vi "Notify Subscribers.vi"(8 "error in (no error)":errorcluster, 9 "Publish Time":timestamp, 10 "Topic Data":variant, 11 "Topic in":refnum<class "Topic.lvclass">) -> (0 "error out":errorcluster, 3 "Topic out":refnum<class "Topic.lvclass">)   [LabVIEW 2015, in "Mediator.lvlib" / "Topic.lvclass"]
doc: "<License>\nCopyright © 2017 Composed Systems, LLC | All rights reserved\nwww.composed.io\n\nAuthor: Ethan Stern <ethan.stern@composed.io>\n\nThis software is provided \"AS IS\" WITHOUT WARRANTIES, either express or implied, AND IS FOR EDUCATIONAL PURPOSES ONLY.\n</License>"
uses:
  Topic.lvclass
  Topic.lvclass/Topic.ctl
  IMediator/SubscriptionRequest/SubscriptionRequest.lvclass
  IMediator/ISubscriptionPolicy/ISubscriptionPolicy.lvclass
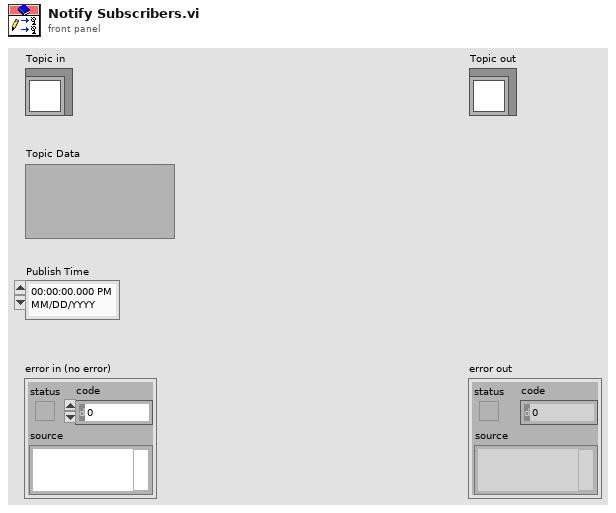
[diagram p1: front panel]
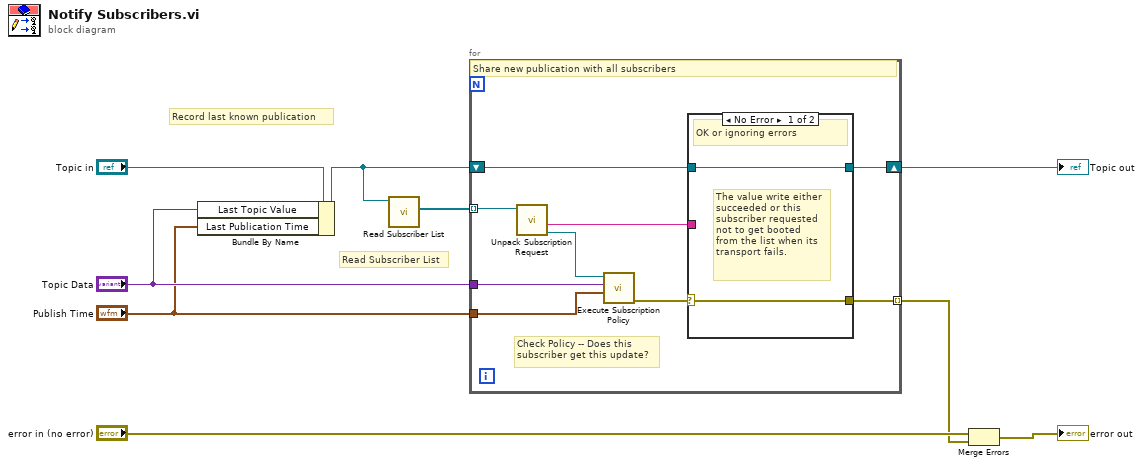
[diagram p0: block diagram]
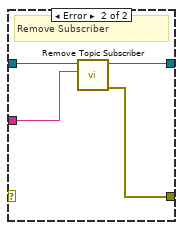
[diagram p2: hidden frame]
diagram:
  # "Read Subscriber List"
  # "Record last known publication"
  n1 = Bundle By Name(cluster="Topic in", "Last Topic Value"="Topic Data", "Last Publication Time"="Publish Time") -> (w2:refnum<class "Topic.lvclass">)
  n2 = call "Read Subscriber List.vi"("Topic in"=w2) -> ("Subscriber List"=w3:refnum<class "SubscriptionRequest.lvclass">[])  [unwired: 10 in]
  n3 = for {
    tunnel: w3 -> [w18] mode=indexing
    tunnel: "Topic Data" -> [w16]
    tunnel: [w17] -> w7 mode=indexing
    tunnel: "Publish Time" -> [w10]
    shift-right: [w14] -> w5
    shift-left: w2 -> [w15]
    # "Check Policy -- Does this\nsubscriber get this update?"
    # "Share new publication with all subscribers"
    n4 = call "Unpack Subscription Request.vi"("SubscriptionRequest in"=w18) -> ("Subscription Policy"=w12:refnum<data-value>, "Unique Subscriber ID"=w13:string)  [unwired: 7 in, 2 out]
    n5 = call "Execute Subscription Policy.vi"("Publish Time"=w10, "New Topic Value"=w16, "Subscription Policy"=w12) -> ("error out"=w11:errorcluster)  [unwired: 8 in]
    n6 = case shown="No Error" w11 {
      selector: w11 -> [w19 _]
      tunnel: [w19 w24] -> w17
      tunnel: w15 -> [w20 w23]
      tunnel: [w20 w22] -> w14
      tunnel: w13 -> [_ w21]
      frame No Error {
        # "The value write either\nsucceeded or this\nsubscriber requested\nnot to get booted\nfrom the list when its\ntransport fails."
        # "OK or ignoring errors"
      }
      frame Error {
        # "Remove Subscriber"
        n7 = call "Remove Topic Subscriber.vi"("Unique Subscriber ID"=w21, "Topic in"=w23) -> ("error out"=w24:errorcluster, "Topic out"=w22:refnum<class "Topic.lvclass">)  [unwired: 8 in]
      }
    }
  }
  "Topic out" <- w5
  n8 = Merge Errors("error in (no error)", w7) -> (→"error out":errorcluster)
